vi "dfd_Compute Interpolated Filter Coefficients.vi"(8 "error in (no error)":errorcluster, 9 "factor":i32, 10 "denominator in":dbl[](array[numeric]), 11 "numerator in":dbl[](array[numeric])) -> (0 "error out":errorcluster, 2 "denominator out":dbl[](array[numeric]), 3 "numerator out":dbl[](array[numeric]))   [LabVIEW 2017, in "NI_DigFilterLicensed.lvlib"]
uses:
  <vilib>/addons/Digital Filter Design/NI_DigFilterLicensed.lvlib
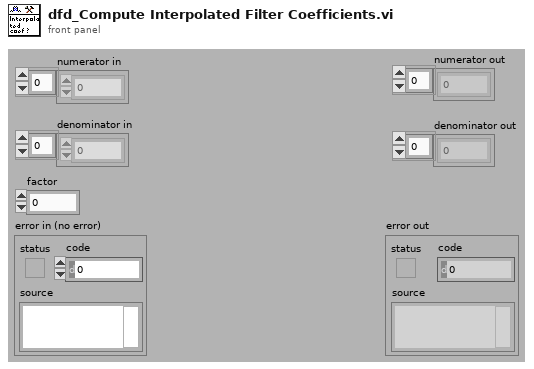
[diagram p1: front panel]
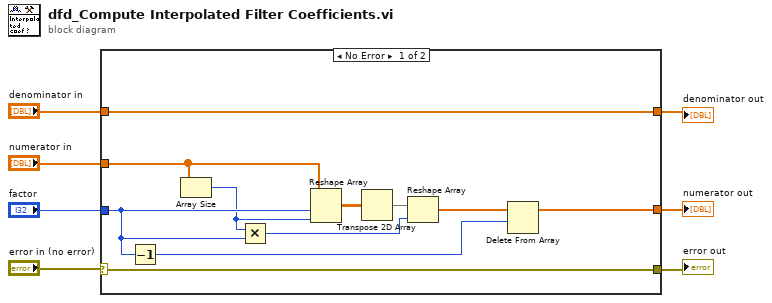
[diagram p0: block diagram]
diagram:
  n1 = case shown="No Error" "error in (no error)" {
    selector: "error in (no error)" -> [w17 w19]
    tunnel: [w13 _] -> w7
    tunnel: "factor" -> [w9 _]
    tunnel: "numerator in" -> [w10 _]
    tunnel: "denominator in" -> [w15 _]
    tunnel: [w15 _] -> w2
    tunnel: [w17 w19] -> w1
    frame No Error {
      n2 = Decrement(x=w9) -> (x-1=w12:i32)
      n3 = Array Size(array=w10) -> (size(s)=w8:i32)
      n4 = Multiply(x=w8, y=w9) -> (x*y=w14:i32)
      n5 = Reshape Array(w10, w9, w8) -> (w11:dbl[][])
      n6 = Transpose 2D Array(2D array=w11) -> (transposed array=w16:dbl[][])
      n7 = Reshape Array(w16, w14) -> (w18:dbl[])
      n8 = Delete From Array(array=w18, length=w12) -> (array with subset deleted=w13:dbl[])  [unwired: 1 in, 1 out]
    }
    frame Error {
    }
  }
  "numerator out" <- w7
  "denominator out" <- w2
  "error out" <- w1
